vi "CopyImagetoTemp.vi"(8 "error in (no error)":errorcluster, 10 "reference":refnum<k7>, 11 "IN":T1={"step name 1"="", "updata 2"="1000", "limitdata 3"="", "load vi name 4"="", "parameter 5"=""}) -> (0 "error out":errorcluster, 2 "reference out":refnum<k7>, 3 "Cluster":T2)   [LabVIEW 2013]
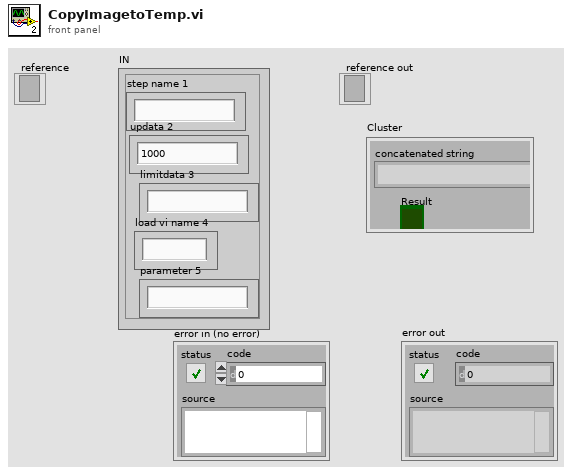
[diagram p1: front panel]
types:
  T1 = cluster{"step name 1":string, "updata 2":string, "limitdata 3":string, "load vi name 4":string, "parameter 5":string}
  T2 = cluster{"concatenated string":string, "Result":bool}
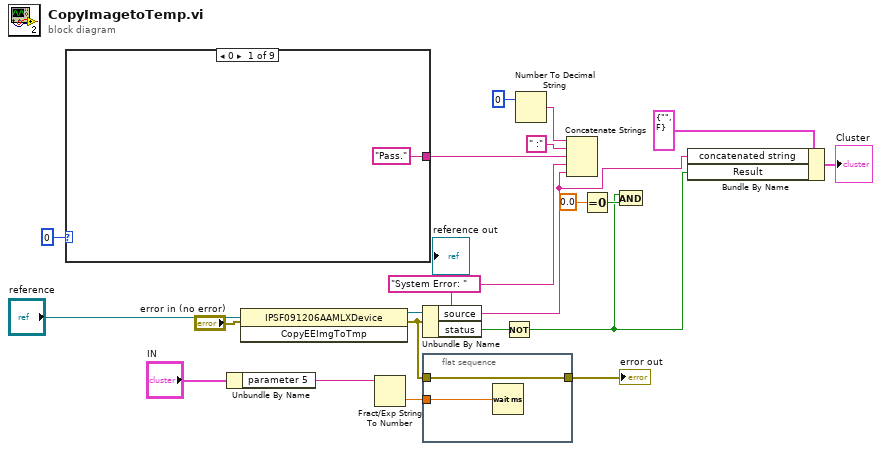
[diagram p0: block diagram]
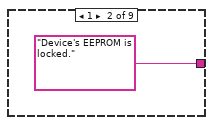
[diagram p2: hidden frame]
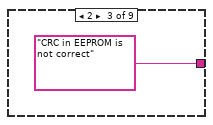
[diagram p3: hidden frame]
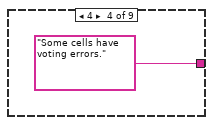
[diagram p4: hidden frame]
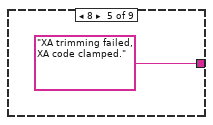
[diagram p5: hidden frame]
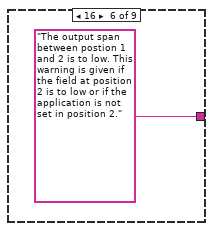
[diagram p6: hidden frame]
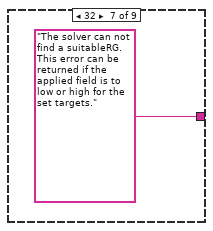
[diagram p7: hidden frame]
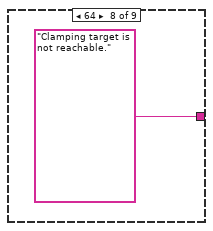
[diagram p8: hidden frame]
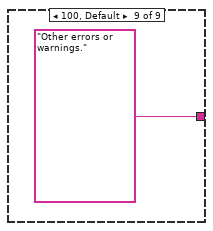
[diagram p9: hidden frame]
diagram:
  n1 = case shown="0" 0 ("ReadFullEepromToImg") {
    tunnel: ["Pass." "Device's EEPROM is locked." "CRC in EEPROM is not correct" "Some cells have voting errors." "XA trimming failed, XA code clamped." "The output span between postion 1 and 2 is to low. This warning is given if the field at position 2 is to low or if the application is not set in position 2." "The solver can not find a suitableRG. This error can be returned if the applied field is to low or high for the set targets." "Clamping target is not reachable." "Other errors or warnings."] -> w14
    frame 0 {
    }
    frame 1 {
    }
    frame 2 {
    }
    frame 4 {
    }
    frame 8 {
    }
    frame 16 {
    }
    frame 32 {
    }
    frame 64 {
    }
    frame 100, Default {
    }
  }
  n2 = Unbundle By Name("IN") -> ("parameter 5"=w17:string)
  n3 = invoke class="IPSF091206AAMLXDevice" method="CopyEEImgToTmp"(reference="reference", error in="error in (no error)") -> (reference out=→"reference out":refnum<k7>, error out=w5:errorcluster)  [unwired: 1 in, 1 out]
  n4 = Fract/Exp String To Number(string=w17) -> (number=w18:dbl)  [unwired: 3 in, 1 out]
  n5 = Unbundle By Name(w5) -> ("source"=w3:string, "status"=w13:bool)
  n6 = flat-sequence {
    tunnel: w18 -> [w32]
    tunnel: w5 -> [w31]
    tunnel: [w31] -> w4
    frame #0 {
      n7 = Wait (ms)(milliseconds to wait=w32) -> ()  [unwired: 1 out]
    }
  }
  n8 = Not(x=w13) -> (.not. x?=w6:bool)
  n9 = Number To Decimal String(number=0) -> (decimal integer string=w16:string)  [unwired: 1 in]
  n10 = Concatenate Strings(w16, " :" ("string"), w14, "System Error: " ("string"), w3) -> ()  [unwired: 1 out]
  n11 = Equal To 0?(x=0.0) -> (x = 0?=w12:bool)
  n12 = And(x=w6, y=w12) -> ()  [unwired: 1 out]
  n13 = Bundle By Name(cluster=T2 {"concatenated string"="", "Result"=FALSE} ("Cluster"), "concatenated string"=w3, "Result"=w6) -> (→"Cluster":T2)
  "error out" <- w4
